vi "PH_VacuumControl.Get and Set Pressures.vi"(0 "i ref in":refnum<vi>, 5 "error in (no error)":errorcluster) -> (14 "i ref out":refnum<vi>, 16 "Status":T1 items=["no info", "off/false/out", "on/true/in", "Failure", "Alarm", "Status 1", "Status 2", "Status 3"], 19 "error out":errorcluster)   [LabVIEW 2014, in "PH_VacuumControl.lvlib"]
doc: "This VI gets the pressure values and sets them to the GUI, to own attributes and publishes the result."
uses:
  PH_VacuumControl.lvlib
  PH_Basics/PH_StatusHandler/PH_StatusHandler.Status.ctl
  instr.lib/AGCxxx/AGCxxx - Driver.lvlib
  CSlibraries-extern/DimLVEvent/LVDimInterface/LVDimInterface.lvlib
  PH_Basics/PH_Common/PH_Common.lvlib
  PH_Basics/PH_StatusHandler/PH_StatusHandler.lvlib
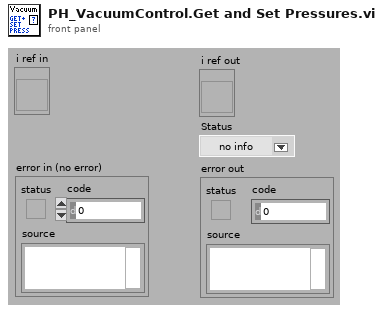
[diagram p1: front panel]
types:
  T1 = typedef "PH_StatusHandler.lvlib/PH_StatusHandler.Status.ctl" = i16
  T2 = typedef "PH_VacuumControl.lvlib/PH_VacuumControl.i attribute.ctl" = cluster{"GUI Refs":cluster{"Exit":refnum<vi>, "Set Unit":refnum<vi>, "Device found":refnum<vi>, "Busy":refnum<vi>, "State":refnum<vi>, "Delete":refnum<vi>, "Channels":refnum<vi>, "Channel Name":refnum<vi>, "Trend":refnum<vi>, "Logarithmic":refnum<vi>, "Limit reached":refnum<vi>, "Channel Name 1 MT":refnum<vi>, "Channel Name 2 MT":refnum<vi>, "Trend MT":refnum<vi>, "Logarithmic MT":refnum<vi>, "Limit reached MT":refnum<vi>}, "Device found":bool, "Busy":bool, "Selected Unit":i32, "Channels [mbar]":T3, "Channel Names":cluster{"Channel 1":string, "Channel 2":string, "Channel 3":string, "Channel 4":string, "Channel 5":string, "Channel 6":string}, "Status":T1, "AGCxxx VISA Cluster":T4, "Instr Firmware Revision":string, "Service IDs Pressure":cluster{"Channel 1":i32, "Channel 2":i32, "Channel 3":i32, "Channel 4":i32, "Channel 5":i32, "Channel 6":i32}, "Service IDs Limits":cluster{"Channel 1":i32, "Channel 2":i32, "Channel 3":i32, "Channel 4":i32, "Channel 5":i32, "Channel 6":i32}, "Trend":cluster{"Start Point":timestamp, "Pressures [mbar] Channel 1":dbl[], "Pressures [mbar] Channel 2":dbl[], "Pressures [mbar] Channel 3":dbl[], "Pressures [mbar] Channel 4":dbl[], "Pressures [mbar] Channel 5":dbl[], "Pressures [mbar] Channel 6":dbl[], "Timebase [s]":i32[], "Trend Channel":u16, "Start Fit":dbl, "Trend Channel 1 MT":u16, "Trend Channel 2 MT":u16, "Start or continue Fit MT":dbl, "Continue or start Fit MT":dbl, "Datasets strored":i32, "Dataarray Size":i32}, "Running":bool}
  T3 = typedef "PH_VacuumControl.lvlib/PH_VacuumControl.Channels.ctl" = cluster{"Channel 1":dbl, "Channel 2":dbl, "Channel 3":dbl, "Channel 4":dbl, "Channel 5":dbl, "Channel 6":dbl, "Name Channel 1":string, "Name Channel 2":string, "Name Channel 3":string, "Name Channel 4":string, "Name Channel 5":string, "Name Channel 6":string, "Upper Limit":dbl, "Upper Limit 2":dbl, "Upper Limit 3":dbl, "Upper Limit 4":dbl, "Upper Limit 5":dbl, "Upper Limit 6":dbl}
  T4 = typedef "AGCxxx - Driver.lvlib/AGCxxx VISA Control.ctl" = cluster{"VISA resource name":refnum<visa-resource-name>, "VISA Timeout Value (1000 ms)":u32, "Lock Timeout (1000 ms)":u32, "MAX Channel (6)":i32}
  T5 = cluster{"Channel 1":string, "Channel 2":string, "Channel 3":string, "Channel 4":string, "Channel 5":string, "Channel 6":string}
  T6 = cluster{"Channel 1":i32, "Channel 2":i32, "Channel 3":i32, "Channel 4":i32, "Channel 5":i32, "Channel 6":i32}
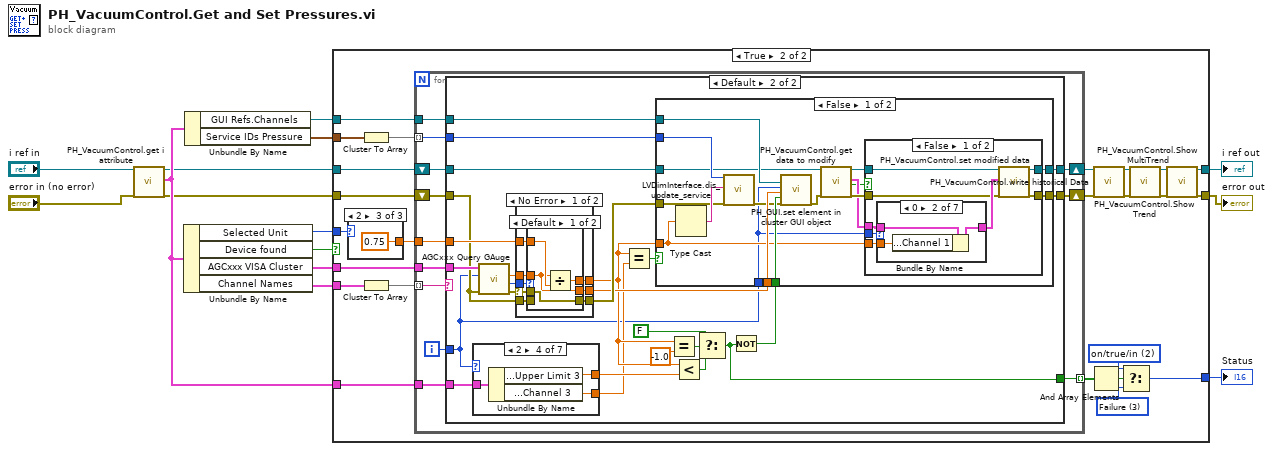
[diagram p0: block diagram]
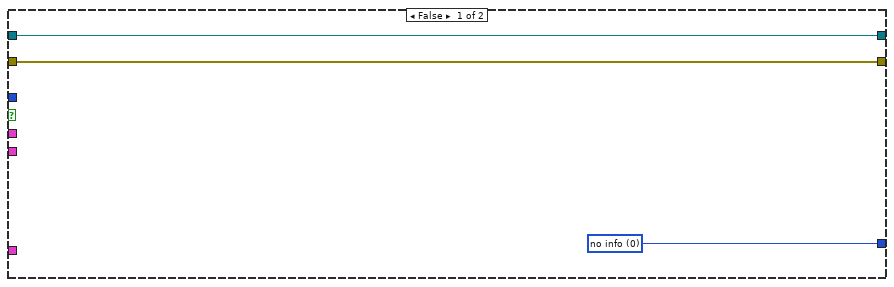
[diagram p2: hidden frame]
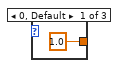
[diagram p3: hidden frame]
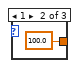
[diagram p4: hidden frame]
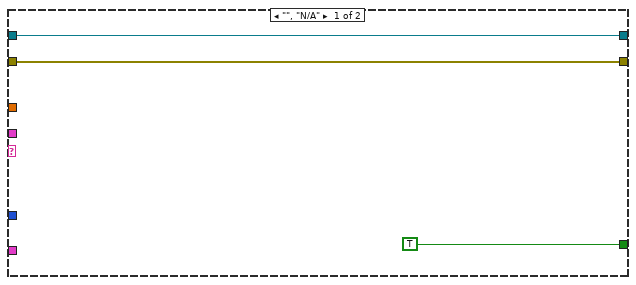
[diagram p5: hidden frame]
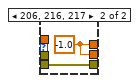
[diagram p6: hidden frame]
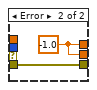
[diagram p7: hidden frame]
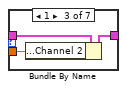
[diagram p9: hidden frame]
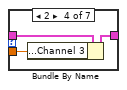
[diagram p10: hidden frame]
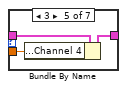
[diagram p11: hidden frame]
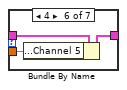
[diagram p12: hidden frame]
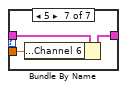
[diagram p13: hidden frame]
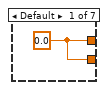
[diagram p16: hidden frame]
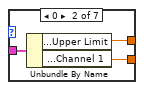
[diagram p17: hidden frame]
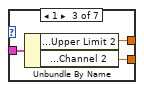
[diagram p18: hidden frame]
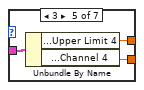
[diagram p19: hidden frame]
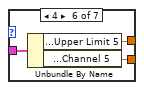
[diagram p20: hidden frame]
diagram:
  n1 = call "PH_VacuumControl.get i attribute.vi"("i ref in"="i ref in", "error in (no error)"="error in (no error)") -> ("i ref out"=w7:refnum<vi>, "i attribute"=w9:T2, "error out"=w8:errorcluster)  [unwired: 15 in]
  n2 = Unbundle By Name(w9) -> ("Selected Unit"=w3:i32, "Device found"=w5:bool, "AGCxxx VISA Cluster"=w6:T4, "Channel Names"=w4:T5)
  n3 = Unbundle By Name(w9) -> ("GUI Refs.Channels"=w1:refnum<vi>, "Service IDs Pressure"=w2:T6)
  n4 = case shown="True" w5 {
    tunnel: w6 -> [_ w41]
    tunnel: [w17 w20] -> w13
    tunnel: w9 -> [_ w27]
    tunnel: w4 -> [_ w40]
    tunnel: w3 -> [_ w38]
    tunnel: w8 -> [w17 w36]
    tunnel: w7 -> [w16 w35]
    tunnel: [w16 w18] -> w12
    tunnel: [w15 w31] -> w14
    tunnel: w2 -> [_ w28]
    tunnel: w1 -> [_ w26]
    frame False {
      w15 = T1 0 items=["no info", "off/false/out", "on/true/in", "Failure", "Alarm", "Status 1", "Status 2", "Status 3"] ("State")
    }
    frame True {
      w32 = T1 2 items=["no info", "off/false/out", "on/true/in", "Failure", "Alarm", "Status 1", "Status 2", "Status 3"] ("State")
      w33 = T1 3 items=["no info", "off/false/out", "on/true/in", "Failure", "Alarm", "Status 1", "Status 2", "Status 3"] ("State")
      n5 = case shown="2" w38 {
        tunnel: [1.0 ("y") 100.0 ("y") 0.75 ("y")] -> w37
        frame 0, Default {
        }
        frame 1 {
        }
        frame 2 {
        }
      }
      n6 = Cluster To Array(cluster=w28) -> (array=w29:i32[])
      n7 = Cluster To Array(cluster=w40) -> (array=w39:string[])
      n8 = for {
        tunnel: w41 -> [w56]
        shift-right: [w54] -> w24
        shift-left: w36 -> [w55]
        tunnel: w39 -> [w47] mode=indexing
        tunnel: w37 -> [w52]
        tunnel: [w51] -> w30 mode=indexing
        shift-right: [w49] -> w25
        shift-left: w35 -> [w50]
        tunnel: w29 -> [w48] mode=indexing
        tunnel: w27 -> [w46]
        tunnel: w26 -> [w45]
        i -> [w53]
        n9 = case shown="Default" w47 {
          tunnel: w56 -> [_ w84]
          tunnel: w55 -> [w59 w73]
          tunnel: [w59 w67] -> w54
          tunnel: w53 -> [_ w61]
          tunnel: w46 -> [_ w66]
          tunnel: w52 -> [_ w81]
          tunnel: [TRUE w65] -> w51
          tunnel: w50 -> [w57 w80]
          tunnel: [w57 w68] -> w49
          tunnel: w48 -> [_ w78]
          tunnel: w45 -> [_ w62]
          frame "", "N/A" {
          }
          frame Default {
            n10 = case shown="2" w61 {
              tunnel: w66 -> [_ w152 w155 w158 w161 w164 w167]
              tunnel: [w149 w151 w154 w157 w160 w163 w166] -> w72
              tunnel: [w149 w150 w153 w156 w159 w162 w165] -> w64
              frame Default {
                w149 = 0.0
              }
              frame 0 {
                n11 = Unbundle By Name(w152) -> ("Channels [mbar].Upper Limit"=w151:dbl, "Channels [mbar].Channel 1"=w150:dbl)
              }
              frame 1 {
                n12 = Unbundle By Name(w155) -> ("Channels [mbar].Upper Limit 2"=w154:dbl, "Channels [mbar].Channel 2"=w153:dbl)
              }
              frame 2 {
                n13 = Unbundle By Name(w158) -> ("Channels [mbar].Upper Limit 3"=w157:dbl, "Channels [mbar].Channel 3"=w156:dbl)
              }
              frame 3 {
                n14 = Unbundle By Name(w161) -> ("Channels [mbar].Upper Limit 4"=w160:dbl, "Channels [mbar].Channel 4"=w159:dbl)
              }
              frame 4 {
                n15 = Unbundle By Name(w164) -> ("Channels [mbar].Upper Limit 5"=w163:dbl, "Channels [mbar].Channel 5"=w162:dbl)
              }
              frame 5 {
                n16 = Unbundle By Name(w167) -> ("Channels [mbar].Upper Limit 6"=w166:dbl, "Channels [mbar].Channel 6"=w165:dbl)
              }
            }
            n17 = call "AGCxxx Query GAuge.vi"("error in (no error)"=w73, "Channel (0)"=w61, "AGCxxx VISA Cluster"=w84) -> ("error out"=w60:errorcluster, "AGC Errno"=w83:i32, "Gauge"=w82:dbl)  [unwired: 5 in, 1 out]
            n18 = case shown="No Error" w60 {
              selector: w60 -> [w85 _]
              tunnel: w83 -> [w92 _]
              tunnel: w82 -> [w91 _]
              tunnel: w81 -> [w90 _]
              tunnel: [w89 w100] -> w79
              tunnel: w73 -> [w88 w100]
              tunnel: [w87 w99] -> w70
              tunnel: [w86 w99] -> w69
              frame No Error {
                n19 = case shown="Default" w92 {
                  tunnel: w91 -> [w93 _]
                  tunnel: [w96 w98] -> w89
                  tunnel: w85 -> [w96 _]
                  tunnel: w88 -> [_ w98]
                  tunnel: [w95 w97] -> w86
                  tunnel: w90 -> [w94 _]
                  tunnel: [w93 w97] -> w87
                  frame Default {
                    n20 = Divide(x=w93, y=w94) -> (x/y=w95:dbl)
                  }
                  frame 206, 216, 217 {
                    w97 = -1.0 ("Gauge")
                  }
                }
              }
              frame Error {
                w99 = -1.0 ("Gauge")
              }
            }
            n21 = Equal?(x=w69, y=w64) -> (x = y?=w63:bool)
            n22 = Equal?(x=w69, y=-1.0) -> (x = y?=w76:bool)
            n23 = Less?(x=w69, y=w72) -> (x < y?=w74:bool)
            n24 = Select(t=FALSE, s=w76, f=w74) -> (s? t:f=w65:bool)
            n25 = Not(x=w65) -> (.not. x?=w71:bool)
            n26 = case shown="False" w63 {
              tunnel: w80 -> [w102 w148]
              tunnel: w79 -> [w101 w147]
              tunnel: w78 -> [w116 _]
              tunnel: w71 -> [w115 _]
              tunnel: w70 -> [w114 _]
              tunnel: w69 -> [w104 _]
              tunnel: [w112 w148] -> w68
              tunnel: [w111 w147] -> w67
              tunnel: w61 -> [w103 _]
              tunnel: w62 -> [w105 _]
              frame False {
                n27 = Type Cast(x=w104) -> (*(type *) &x=w117:string)  [unwired: 1 in]
                n28 = call "LVDimInterface.dis_update_service.vi"("my_serviceID"=w116, "data"=w117, "error in (no error)"=w101) -> ("error out"=w113:errorcluster)  [unwired: 14 in, 2 out]
                n29 = call "PH_GUI.set element in cluster GUI object.vi"("Cluster Ref"=w105, "Cluster index"=w103, "Value"=w114, "Blinking? (false)"=w115, "error in (no error)"=w113) -> ("error out"=w110:errorcluster)  [unwired: 14 in]
                n30 = call "PH_VacuumControl.get data to modify.vi"("i ref in"=w102, "error in (no error)"=w110) -> ("i ref out"=w109:refnum<vi>, "i attribute"=w107:T2, "timed out"=w106:bool, "error out"=w108:errorcluster)  [unwired: 14 in]
                n31 = case shown="False" w106 {
                  tunnel: w104 -> [w125 _]
                  tunnel: [w123 w146] -> w112
                  tunnel: [w122 w145] -> w111
                  tunnel: w109 -> [w121 w146]
                  tunnel: w108 -> [w120 w145]
                  tunnel: w107 -> [w119 _]
                  tunnel: w103 -> [w118 _]
                  frame False {
                    n32 = case shown="0" w118 {
                      tunnel: w119 -> [w126 w127 w130 w134 w137 w140 w143]
                      tunnel: [w126 w129 w132 w135 w138 w141 w144] -> w124
                      tunnel: w125 -> [_ w128 w131 w133 w136 w139 w142]
                      frame Default {
                      }
                      frame 0 {
                        n33 = Bundle By Name(cluster=w127, "Channels [mbar].Channel 1"=w128) -> (w129:T2)
                      }
                      frame 1 {
                        n34 = Bundle By Name(cluster=w130, "Channels [mbar].Channel 2"=w131) -> (w132:T2)
                      }
                      frame 2 {
                        n35 = Bundle By Name(cluster=w134, "Channels [mbar].Channel 3"=w133) -> (w135:T2)
                      }
                      frame 3 {
                        n36 = Bundle By Name(cluster=w137, "Channels [mbar].Channel 4"=w136) -> (w138:T2)
                      }
                      frame 4 {
                        n37 = Bundle By Name(cluster=w140, "Channels [mbar].Channel 5"=w139) -> (w141:T2)
                      }
                      frame 5 {
                        n38 = Bundle By Name(cluster=w143, "Channels [mbar].Channel 6"=w142) -> (w144:T2)
                      }
                    }
                    n39 = call "PH_VacuumControl.set modified data.vi"("i ref in"=w121, "i attribute"=w124, "error in (no error)"=w120) -> ("i ref out"=w123:refnum<vi>, "error out"=w122:errorcluster)  [unwired: 15 in]
                  }
                  frame True {
                  }
                }
              }
              frame True {
              }
            }
          }
        }
      }
      n40 = And Array Elements(Boolean array=w30) -> (logical AND=w34:bool)
      n41 = call "PH_VacuumControl.write historical Data.vi"("i ref in"=w25, "error in"=w24) -> ("i ref out"=w21:refnum<vi>, "error out"=w22:errorcluster)  [unwired: 16 in]
      n42 = Select(t=w32, s=w34, f=w33) -> (s? t:f=w31:T1)
      n43 = call "PH_VacuumControl.Show Trend.vi"("i ref in"=w21, "error in"=w22) -> ("i ref out"=w19:refnum<vi>, "error out"=w23:errorcluster)  [unwired: 16 in]
      n44 = call "PH_VacuumControl.Show MultiTrend.vi"("i ref in"=w19, "error in"=w23) -> ("i ref out"=w18:refnum<vi>, "error out"=w20:errorcluster)  [unwired: 16 in]
    }
  }
  "Status" <- w14
  "error out" <- w13
  "i ref out" <- w12
